vi "Theta Drive_Two step on.vi"(9 "Start Location Step (-90to90)":i32, 10 "Target Step (-90to90)":i32, 11 "stop":bool) -> (1 "Current Motor Step (0to3)":i32, 2 "Current Step (-90to90)":i32, 3 "Boolean array":bool[](array[boolean]))   [LabVIEW 2017]
uses:
  <vilib>/myRIO/Common/Instrument Driver Framework/myRIO v1.0/DIO/typedefs/DIO Channels Enum.ctl
  <vilib>/myRIO/Common/Instrument Driver Framework/myRIO v1.0/DIO/typedefs/DIO Channels List.ctl
  <vilib>/myRIO/Common/Instrument Driver Framework/Utilities/typedefs/Generic FPGA Reference.ctl
  <vilib>/myRIO/Common/Instrument Driver Framework/Utilities/typedefs/myRIO v1.0 Reference.ctl
  <vilib>/myRIO/Common/Instrument Driver Framework/Utilities/typedefs/Hardware Version Enum.ctl
  <vilib>/myRIO/Common/Instrument Driver Framework/Utilities/typedefs/myRIO Generic Hardware Reference.ctl
  <vilib>/myRIO/Instrument Drivers/Onboard IO/DIO/typedefs/DIO Reference.ctl
  <vilib>/myRIO/Instrument Drivers/Onboard IO/DIO/vis/Write.vi
  <vilib>/userdefined/High Color/nirio_resource_hc.ctl
  <vilib>/myRIO/Common/Instrument Driver Framework/myRIO v1.0/DIO/vis/myRIO v1.1 Open DIO.vi
  <vilib>/myRIO/Instrument Drivers/Onboard IO/DIO/vis/myRIO DIO Open.xnode
  <vilib>/myRIO/Common/Instrument Driver Framework/Utilities/vis/Is FPGA Ref Available.vi
  <vilib>/myRIO/Express VI/Onboard IO/DO/DO Express VI.xnode
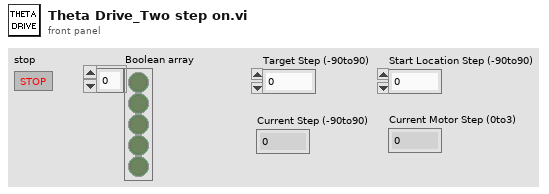
[diagram p1: front panel]
types:
  T1 = typedef "DIO.lvlib/DIO Reference.ctl" = cluster{"myRIO Reference":T2, "DIO Channels List":T6}
  T2 = typedef "myRIO Generic Hardware Reference.ctl" = cluster{"myRIO Model":T3, "myRIO Hardware Reference":T4}
  T3 = typedef "Hardware Version Enum.ctl" = enum16{"Unknown", "myRIO-1900", "myRIO-1950", "roboRIO", "NI ELVIS RIO CM"}
  T4 = typedef "myRIO v1.0 Reference.ctl" = cluster{"Generic FPGA Reference":T5, "Allow multiple opens":bool}
  T5 = typedef "Generic FPGA Reference.ctl" = refnum<k20>
  T6 = typedef "DIO Channels List.ctl" = T7[]
  T7 = typedef "DIO Channels Enum.ctl" = enum16{"Not Connected", "C/DIO0", "C/DIO1", "C/DIO2", "C/DIO3", "C/DIO4", "C/DIO5", "C/DIO6", "C/DIO7", "A/DIO0", "A/DIO1", "A/DIO2", "A/DIO3", "A/DIO4", "A/DIO5", "A/DIO6", "A/DIO7", "A/DIO8", "A/DIO9", "A/DIO10", "A/DIO11", "A/DIO12", "A/DIO13", "A/DIO14", "A/DIO15", "B/DIO0", "B/DIO1", "B/DIO2", "B/DIO3", "B/DIO4", "B/DIO5", "B/DIO6", "B/DIO7", "B/DIO8", "B/DIO9", "B/DIO10", "B/DIO11", "B/DIO12", "B/DIO13", "B/DIO14", "B/DIO15", "LED0", "LED1", "LED2", "LED3", "Button0", "DIO/DIO0", "DIO/DIO1", "DIO/DIO2", "DIO/DIO3", "DIO/DIO4", "DIO/DIO5", "DIO/DIO6", "DIO/DIO7", "DIO/DIO8", "DIO/DIO9", "SPI/CS0", "SPI/CS1", "SPI/CS2", "SPI/CS3", "LED RADIO (Green)", "LED RADIO (Red)", "LED COMM (Green)", "LED COMM (Red)", "LED MODE (Green)", "LED MODE (Red)"}
  T8 = typedef "nirio_resource_hc.ctl" = tag
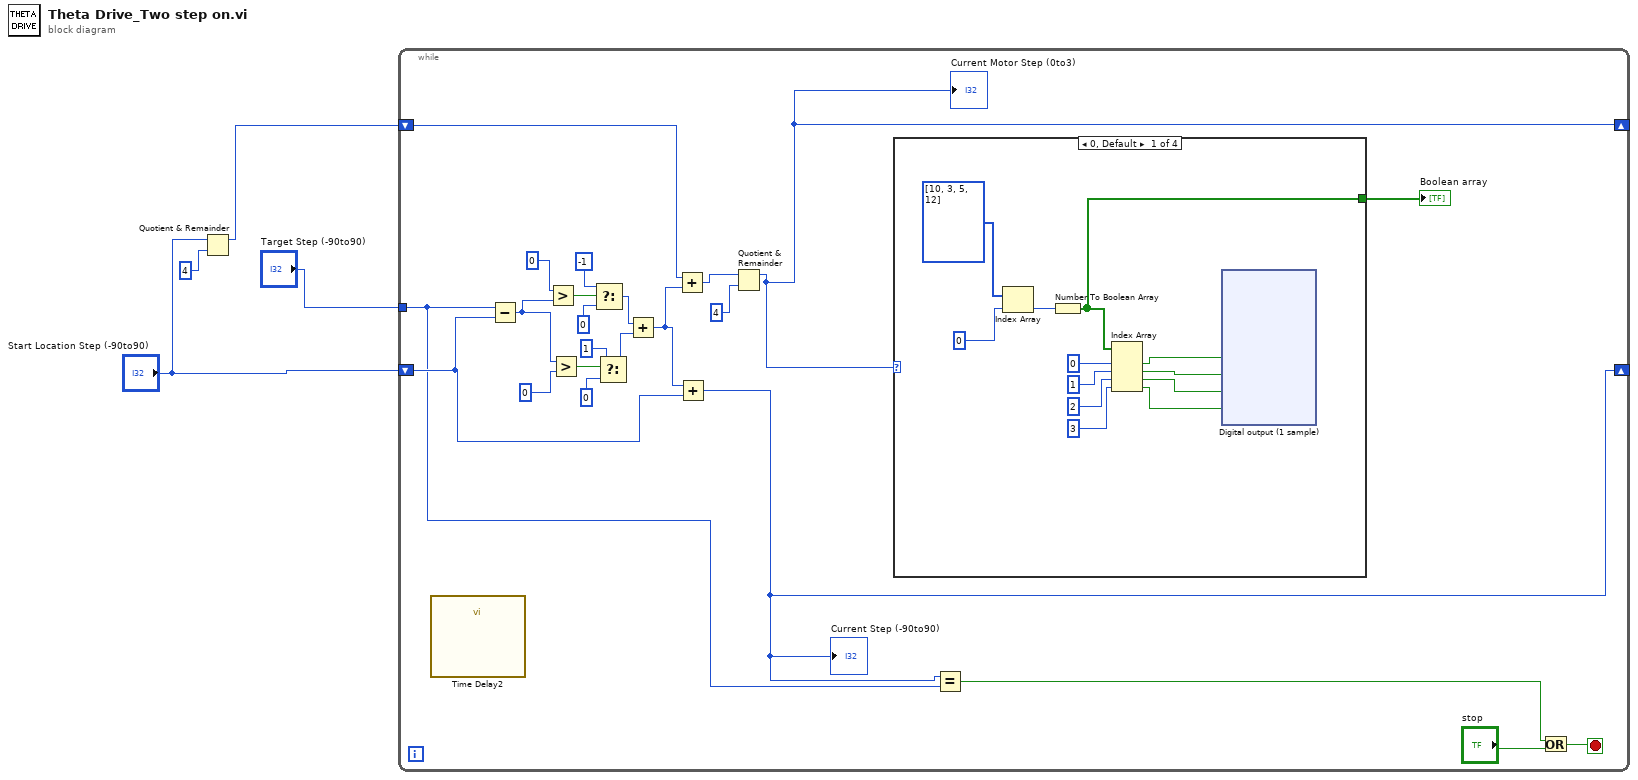
[diagram p0: block diagram]
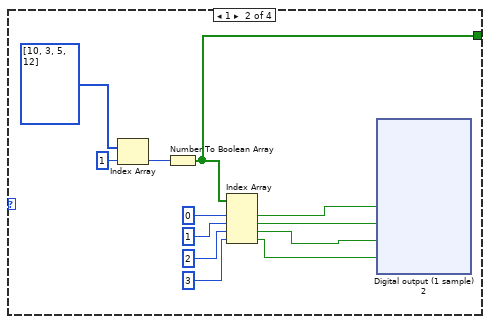
[diagram p2: hidden frame]
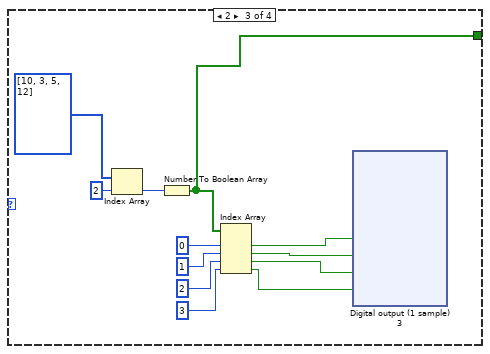
[diagram p3: hidden frame]
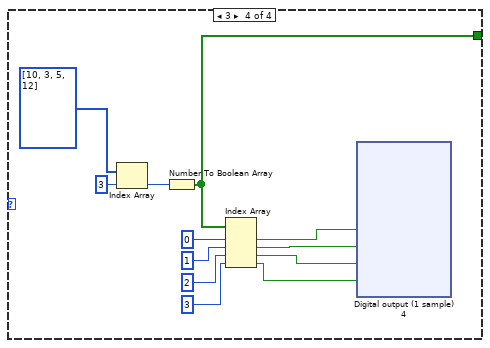
[diagram p4: hidden frame]
diagram:
  n1 = Quotient & Remainder(x="Start Location Step (-90to90)", y=4) -> (x-y*floor(x/y)=w1:i32)  [unwired: 1 out]
  n2 = while {
    shift-right: [w9] -> _
    shift-left: "Start Location Step (-90to90)" -> [w10]
    tunnel: "Target Step (-90to90)" -> [w8]
    shift-right: [w12] -> _
    shift-left: w1 -> [w13]
    stop <- w7 stop-if-true
    n3 = call "Time Delay2"() -> ()  [unwired: 11 in, 1 out]
    n4 = Subtract(x=w8, y=w10) -> (x-y=w25:i32)
    n5 = Greater?(x=0, y=w25) -> (0:w23:bool)
    n6 = Greater?(x=w25, y=0) -> (0:w20:bool)
    n7 = Select(t=-1, s=w23, f=0) -> (s? t:f=w17:i32)
    n8 = Select(t=1, s=w20, f=0) -> (s? t:f=w16:i32)
    n9 = Add(x=w17, y=w16) -> (x+y=w11:i32)
    n10 = Add(x=w13, y=w11) -> (x+y=w15:i32)
    n11 = Add(x=w11, y=w10) -> (x+y=w9:i32)
    "Current Step (-90to90)" <- w9
    n12 = Quotient & Remainder(x=w15, y=4) -> (x-y*floor(x/y)=w12:i32)  [unwired: 1 out]
    "Current Motor Step (0to3)" <- w12
    n13 = case shown="0, Default" w12 {
      tunnel: [w35 w80 w129 w179] -> w27
      frame 0, Default {
        n14 = Index Array(array=i32[] [10, 3, 5, 12], index=0) -> (element=w34:i32)
        n15 = Number To Boolean Array(number=w34) -> (Boolean array=w35:bool[])
        n16 = Index Array(array=w35, index #1=0 ("index"), index #2=1 ("index"), index #3=2 ("index"), index #4=3 ("index")) -> (element #1=w31:bool, element #2=w30:bool, element #3=w29:bool, element #4=w28:bool)
        n17 = xnode "Digital output (1 sample)"("A/DIO0 (Pin 11)"=w31, "A/DIO1 (Pin 13)"=w30, "A/DIO2 (Pin 15)"=w29, "A/DIO3 (Pin 17)"=w28) -> ()  [unwired: 1 in, 1 out]
      }
      frame 1 {
        n18 = Index Array(array=i32[] [10, 3, 5, 12], index=1) -> (element=w81:i32)
        n19 = Number To Boolean Array(number=w81) -> (Boolean array=w80:bool[])
        n20 = Index Array(array=w80, index #1=0 ("index"), index #2=1 ("index"), index #3=2 ("index"), index #4=3 ("index")) -> (element #1=w89:bool, element #2=w88:bool, element #3=w87:bool, element #4=w86:bool)
        n21 = xnode "Digital output (1 sample) 2"("A/DIO0 (Pin 11)"=w89, "A/DIO1 (Pin 13)"=w88, "A/DIO2 (Pin 15)"=w87, "A/DIO3 (Pin 17)"=w86) -> ()  [unwired: 1 in, 1 out]
      }
      frame 2 {
        n22 = Index Array(array=i32[] [10, 3, 5, 12], index=2) -> (element=w131:i32)
        n23 = Number To Boolean Array(number=w131) -> (Boolean array=w129:bool[])
        n24 = Index Array(array=w129, index #1=0 ("index"), index #2=1 ("index"), index #3=2 ("index"), index #4=3 ("index")) -> (element #1=w139:bool, element #2=w138:bool, element #3=w137:bool, element #4=w136:bool)
        n25 = xnode "Digital output (1 sample) 3"("A/DIO0 (Pin 11)"=w139, "A/DIO1 (Pin 13)"=w138, "A/DIO2 (Pin 15)"=w137, "A/DIO3 (Pin 17)"=w136) -> ()  [unwired: 1 in, 1 out]
      }
      frame 3 {
        n26 = Index Array(array=i32[] [10, 3, 5, 12], index=3) -> (element=w181:i32)
        n27 = Number To Boolean Array(number=w181) -> (Boolean array=w179:bool[])
        n28 = Index Array(array=w179, index #1=0 ("index"), index #2=1 ("index"), index #3=2 ("index"), index #4=3 ("index")) -> (element #1=w189:bool, element #2=w188:bool, element #3=w187:bool, element #4=w186:bool)
        n29 = xnode "Digital output (1 sample) 4"("A/DIO0 (Pin 11)"=w189, "A/DIO1 (Pin 13)"=w188, "A/DIO2 (Pin 15)"=w187, "A/DIO3 (Pin 17)"=w186) -> ()  [unwired: 1 in, 1 out]
      }
    }
    "Boolean array" <- w27
    n30 = Equal?(x=w9, y=w8) -> (x = y?=w5:bool)
    n31 = Or(x=w5, y="stop") -> (x .or. y?=w7:bool)
  }
